vi "Watson.vi"() -> ()   [LabVIEW 2019]
uses:
  Program Files (x86)/National Instruments/LabVIEW 2019/project/EN1Course-master (12)/EN1Course-master/_Subs/ThingWorx/_TW_Subs/TW_XControl.xctl
  Program Files (x86)/National Instruments/LabVIEW 2019/project/EN1Course-master (12)/EN1Course-master/_Subs/ThingWorx/_TW_Subs/Thingworx_Write_string.vi
  <vilib>/httpClient/POSTBuffer.vi
  <vilib>/httpClient/LabVIEWHTTPClient.lvlib
panel:
  in  "Thingwork":string(xcontrol)
  in  "url 2":string="http://172.16.148.158"
  in  "url":string="http://172.16.148.158"
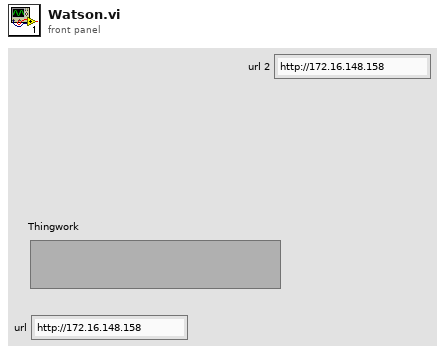
[diagram p1: front panel]
types:
  T1 = typedef "imagedata.ctl" = cluster{"image type":i32, "image depth":i32, "image":u8[], "mask":u8[], "colors":u32[], "Rectangle":cluster{"left":i16, "top":i16, "right":i16, "bottom":i16}}
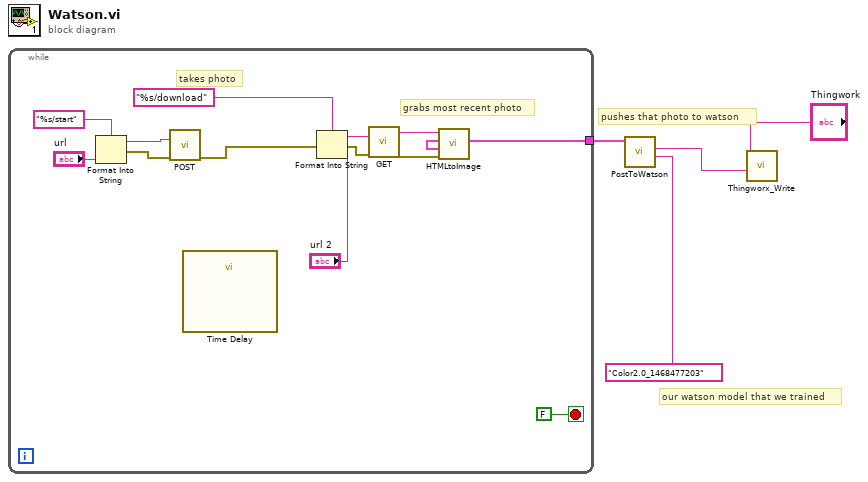
[diagram p0: block diagram]
diagram:
  # "our watson model that we trained"
  # "pushes that photo to watson"
  n1 = while {
    tunnel: [w11] -> w3
    stop <- FALSE stop-if-true
    # "grabs most recent photo"
    # "takes photo"
    n2 = Format Into String(format string="%s/start" ("url"), "url") -> (resulting string=w17:string, error out=w6:errorcluster)  [unwired: 2 in]
    n3 = call-poly <vilib>:"POST.vi"("url"=w17, "error in (no error)"=w6) -> ("error out"=w7:errorcluster)  [unwired: 10 in, 3 out]
    n4 = call "Time Delay"() -> ()  [unwired: 11 in, 1 out]
    n5 = Format Into String(format string="%s/download" ("url"), error in=w7, "url 2") -> (resulting string=w12:string, error out=w5:errorcluster)  [unwired: 1 in]
    n6 = call <vilib>:"GET.vi"("url"=w12, "error in (no error)"=w5) -> ("body"=w15:string, "error out"=w14:errorcluster)  [unwired: 10 in, 2 out]
    n7 = call "HTMLtoImage.vi"("error in (no error)"=w14, "body"=w15) -> ("image data"=w11:T1)  [unwired: 8 in, 1 out]
  }
  n8 = call "PostToWatson.vi"("Model Name"="Color2.0_1468477203", "image in"=w3) -> ("class"=w2:string)  [unwired: 5 in, 4 out]
  n9 = call-poly "Thingworx_Write.vi"("String"=w2, "Thingworx"="Thingwork") -> ()  [unwired: 10 in]
